vi "Main Test Program.vi"() -> ()   [LabVIEW 2014]
panel:
  in  "Version Sheet Cluster":T1={"Folder Path containing version information"=path "C:/Version", "File name (including .ini)"=path "version sheet.ini", "Section"="Utility"}
  out "current time":timestamp
  out "ini file path":path
  in  "stop":bool
  # "Main Program"
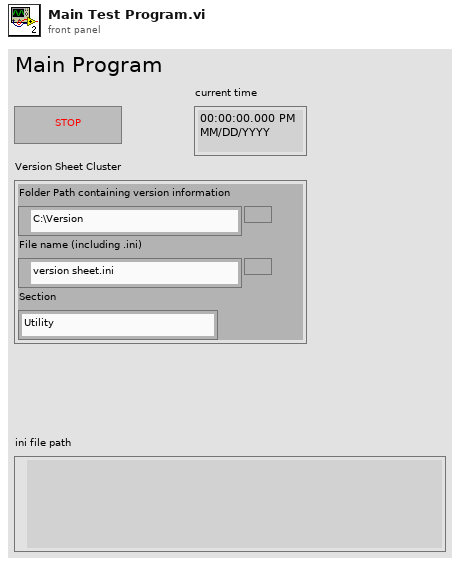
[diagram p1: front panel]
types:
  T1 = cluster{"Folder Path containing version information":path, "File name (including .ini)":path, "Section":string}
  T2 = cluster{"Current VI's Path":path, "This VI ref":refnum<vi>, "Application Level":u8}
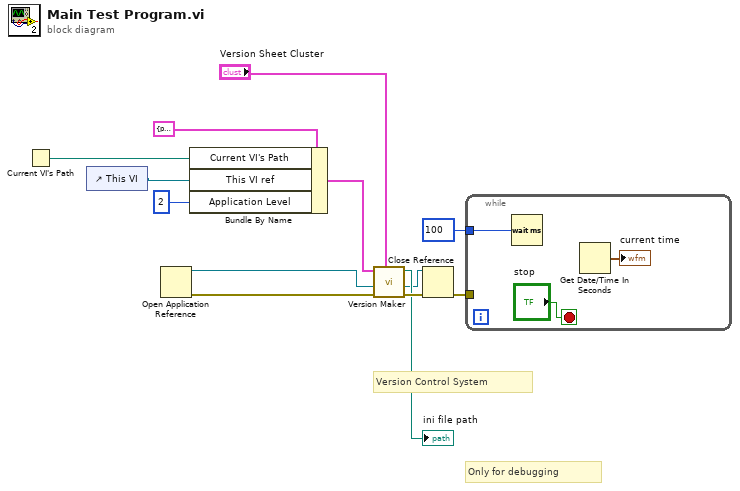
[diagram p0: block diagram]
diagram:
  # "Only for debugging"
  # "Version Control System"
  n1 = Current VI's Path() -> (path=w5:path)
  n2 = control-ref of="This VI"() -> (w4:refnum<vi>)
  n3 = Open Application Reference() -> (0:w12:errorcluster, 3:w9:refnum<vi>)  [unwired: 4 in]
  n4 = Bundle By Name(cluster=T2 {"Current VI's Path"=path "C:/Ehsan Temp Folder/TFS/Change Management Tool/Files/Main Files/Update Registry.vi", "This VI ref"=refnum, "Application Level"=2} ("VI Information"), "Current VI's Path"=w5, "This VI ref"=w4, "Application Level"=u8 2) -> (w2:T2)
  n5 = call "Version Maker.vi"("Version Sheet Cluster"="Version Sheet Cluster", "Error In"=w12, "Open Application Reference in"=w9, "VI Information"=w2) -> ("Error Out"=w11:errorcluster, "Open Application Reference out"=w8:refnum<vi>, "ini file path"=→"ini file path":path)  [unwired: 4 in, 1 out]
  n6 = Close Reference(reference=w8, error in (no error)=w11) -> (error out=w7:errorcluster)
  n7 = while {
    tunnel: u32 100 ("milliseconds to wait") -> [w15]
    tunnel: w7 -> [_]
    stop <- "stop" stop-if-true
    n8 = Wait (ms)(milliseconds to wait=w15) -> ()  [unwired: 1 out]
    n9 = Get Date/Time In Seconds() -> (seconds since 1Jan1904=→"current time":timestamp)
  }
